vi "SUB_Chk_RelaySASB.vi"() -> (0 "Relay Board Type":string, 1 "Find?":bool)   [LabVIEW 2011]
uses:
  <vilib>/DAQmx/create/channels.llb/DAQmx Create Channel (DI-Digital Input).vi
  <vilib>/DAQmx/read.llb/DAQmx Read (Digital 1D Bool NChan 1Samp 1Line).vi
panel:
  out "data":bool[](array[boolean])
  out "Device Name":string
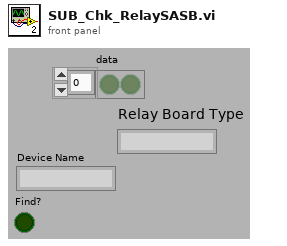
[diagram p1: front panel]
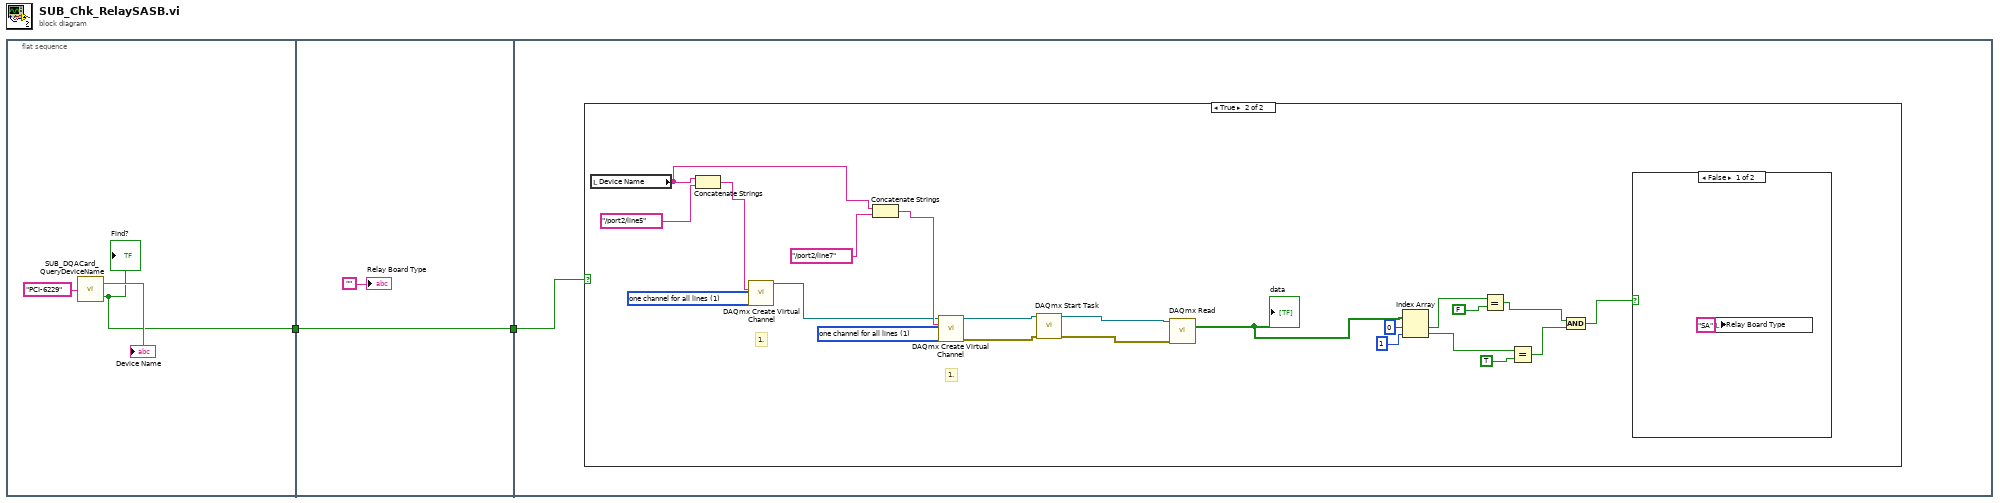
[diagram p0: block diagram]
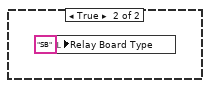
[diagram p3: hidden frame]
diagram:
  n1 = flat-sequence {
    tunnel: [w3] -> w1
    tunnel: [w6] -> w2
    tunnel: w1 -> [w6]
    tunnel: w2 -> [w8]
    frame #0 {
      n2 = call "SUB_DQACard_QueryDeviceName.vi"("Search device type"="PCI-6229") -> ("Device Name"=→"Device Name":string, "Find?"=w3:bool)
      "Find?" <- w3
    }
    frame #1 {
      "Relay Board Type" <- ""
    }
    frame #2 {
      n3 = case shown="True" w8 {
        frame False {
        }
        frame True {
          w27 = 1 items=["one channel for each line", "one channel for all lines"] ("line grouping")
          w30 = 1 items=["one channel for each line", "one channel for all lines"] ("line grouping")
          # "1."
          # "1."
          n4 = local read "Device Name"() -> (w25:string)
          n5 = Concatenate Strings(w25, "/port2/line5") -> (w28:string)
          n6 = call-poly <vilib>:"DAQmx Create Virtual Channel.vi"("lines"=w28, "line grouping"=w30) -> ("task out"=w23:refnum<k21>)  [unwired: 12 in, 1 out]
          n7 = Concatenate Strings(w25, "/port2/line7") -> (w24:string)
          n8 = call-poly <vilib>:"DAQmx Create Virtual Channel.vi"("task in"=w23, "lines"=w24, "line grouping"=w27) -> ("task out"=w22:refnum<k21>, "error out"=w21:errorcluster)  [unwired: 11 in]
          n9 = call <vilib>:"DAQmx Start Task.vi"("task/channels in"=w22, "error in"=w21) -> ("task out"=w20:refnum<k21>, "error out"=w19:errorcluster)  [unwired: 12 in]
          n10 = call-poly <vilib>:"DAQmx Read.vi"("task/channels in"=w20, "error in"=w19) -> ("data"=w18:bool[])  [unwired: 11 in, 2 out]
          "data" <- w18
          n11 = Index Array(array=w18, index #1=0 ("index"), index #2=1 ("index")) -> (element #1=w15:bool, element #2=w12:bool)
          n12 = Equal?(x=w15, y=FALSE) -> (x = y?=w11:bool)
          n13 = Equal?(x=w12, y=TRUE) -> (x = y?=w10:bool)
          n14 = And(x=w11, y=w10) -> (x .and. y?=w9:bool)
          n15 = case shown="False" w9 {
            frame False {
              n16 = local write "Relay Board Type"("SA" ("Relay Board Type")) -> ()
            }
            frame True {
              n17 = local write "Relay Board Type"("SB" ("Relay Board Type")) -> ()
            }
          }
        }
      }
    }
  }
